vi "PopupWindowCaller.vi"() -> ()   [LabVIEW 2012]
uses:
  <resource>/importtools/Common/Event/NISAST Event.lvclass
panel:
  out "Event out":refnum<class "NISAST Event.lvclass">
  out "LED":bool
  out "波形图表":dbl(graph)
  in  "停止按钮":bool
  in  "窗口弹出":bool
  # "1.运行本VI;\n2.单击窗口弹出, 在弹出窗口中点击\"确定\"或\"取消\";\n3.观察本面板上LED的亮灭情况."
  # "本程序实现的是弹出窗口不阻碍前面板数据更新的功能."
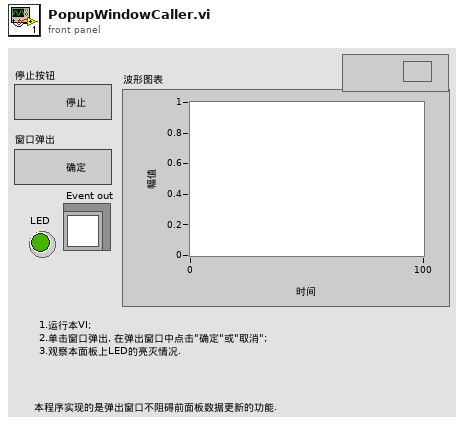
[diagram p1: front panel]
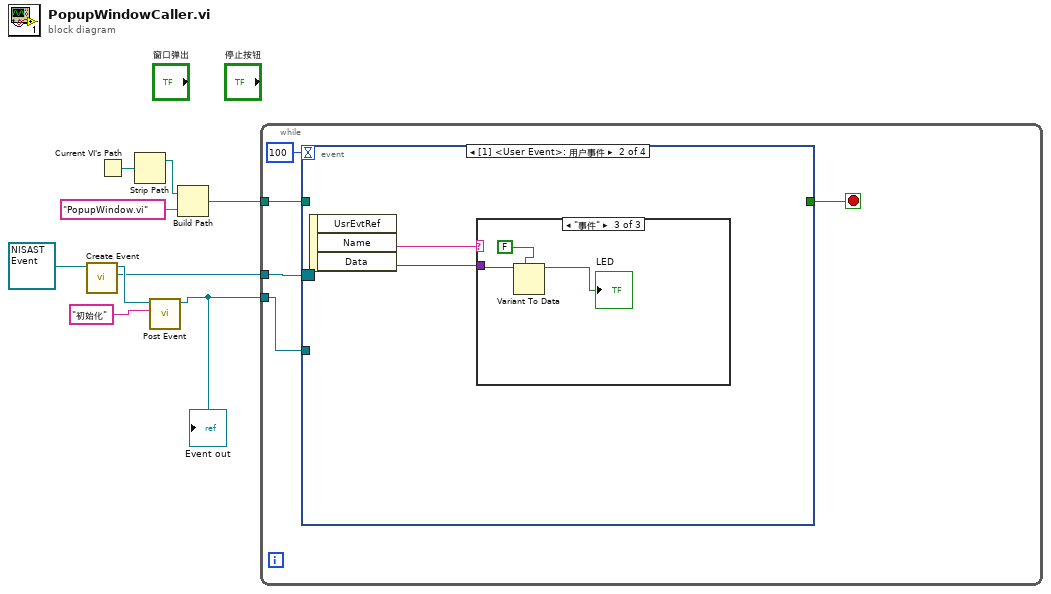
[diagram p0: block diagram]
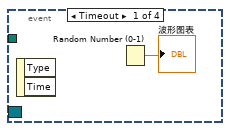
[diagram p2: hidden frame]
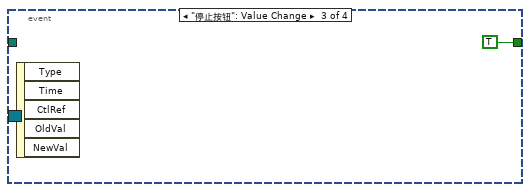
[diagram p5: hidden frame]
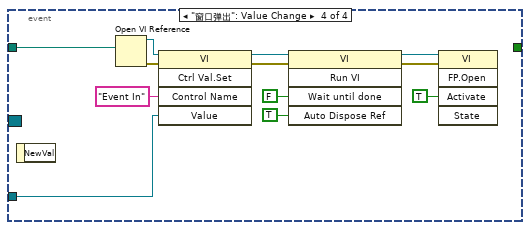
[diagram p6: hidden frame]
diagram:
  n1 = call-dynamic "Create Event.vi"("Event in"=refnum<class "NISAST Event.lvclass"> refnum ("NISAST Event.lvclass")) -> ("Event Registration Refnum"=w1:refnum<event-registration>, "Event out"=w4:refnum<class "NISAST Event.lvclass">)  [unwired: 8 in, 1 out]
  n2 = Current VI's Path() -> (path=w9:path)
  n3 = Strip Path(path=w9) -> (stripped path=w8:path)  [unwired: 1 out]
  n4 = call-dynamic "Post Event.vi"("Event Name"="初始化", "Event in"=w4) -> ("Event out"=w2:refnum<class "NISAST Event.lvclass">)  [unwired: 8 in, 1 out]
  "Event out" <- w2
  n5 = Build Path(base path=w8, name or relative path="PopupWindow.vi" ("名称或相对路径")) -> (appended path=w6:path)
  n6 = while {
    tunnel: w6 -> [w14]
    tunnel: w2 -> [w10]
    tunnel: w1 -> [w11]
    stop <- w13 stop-if-true
    n7 = event shown="[1] <User Event>: 用户事件" {
      selector: w11 -> [_ _ _ _]
      dyn-events: _ -> [_ _ _ _]
      timeout: 100 -> [_ _ _ _]
      tunnel: w14 -> [_ _ _ w33]
      tunnel: [_ _ TRUE _] -> w13
      tunnel: w10 -> [_ _ _ w22]
      event Timeout {
        n8 = event-data() -> ()  [unwired: 1 in, 2 out]
        n9 = Random Number (0-1)() -> (number: 0 to 1=→"波形图表":dbl)
      }
      event User Event {
        n10 = event-data() -> ("Name"=w17:string, "Data"=w16:variant)  [unwired: 1 in, 1 out]
        n11 = case shown="\"事件\"" w17 {
          tunnel: w16 -> [_ _ w20]
          frame "结束", Default {
          }
          frame "初始化" {
          }
          frame "事件" {
            n12 = Variant To Data(type=FALSE, Variant=w20) -> (data=→"LED":bool)  [unwired: 1 in, 1 out]
          }
        }
      }
      event "停止按钮": Value Change {
        n13 = event-data() -> ()  [unwired: 1 in, 5 out]
      }
      event "窗口弹出": Value Change {
        n14 = event-data() -> ()  [unwired: 1 in, 1 out]
        n15 = Open VI Reference(vi path=w33) -> (vi reference=w28:refnum<vi>, error out=w25:errorcluster)  [unwired: 5 in]
        n16 = invoke class="VI" method="Ctrl Val.Set"(reference=w28, error in=w25, "Control Name"="Event In" ("控件名"), "Value"=w22) -> (reference out=w27:refnum<vi>, error out=w24:errorcluster)  [unwired: 1 in, 3 out]
        n17 = invoke class="VI" method="Run VI"(reference=w27, error in=w24, "Wait until done"=FALSE ("结束前等待"), "Auto Dispose Ref"=TRUE ("自动销毁引用")) -> (reference out=w31:refnum<vi>, error out=w30:errorcluster)  [unwired: 1 in, 3 out]
        n18 = invoke class="VI" method="FP.Open"(reference=w31, error in=w30, "Activate"=TRUE ("激活？")) -> ()  [unwired: 2 in, 5 out]
      }
    }
  }
